vi "CLD 13 Flow Rates Solution.vi"() -> ()   [LabVIEW 2014]
doc: "CLD-Lösung 13. Ereignisgesteuerte Zustandsautomatenarchitektur. Die Reihenfolge der Schritte richtet sich nach den Benutzereingaben."
uses:
  CLD 13 State Machine Enum.ctl
  CLD 13 Data Cluster.ctl
  CLD 13 timer Enum.ctl
panel:
  out "Fehler (Ausgang)":errorcluster
  in  "Fehler (Eingang, kein Fehler)":errorcluster
  out "Durchflussmesser":i8(knob) scale=-20.0..20.0 scale format="%_2f"
  in  "Applikation stoppen":bool
  in  "Durchfluss stoppen":bool
  out "Verstrichene Zeit":dbl format="%#.1g"
  out "Flussrate":dbl
  in  "Flussratenänderung":i8(slide) min=-2 max=2 step=1 scale=-2.0..2.0
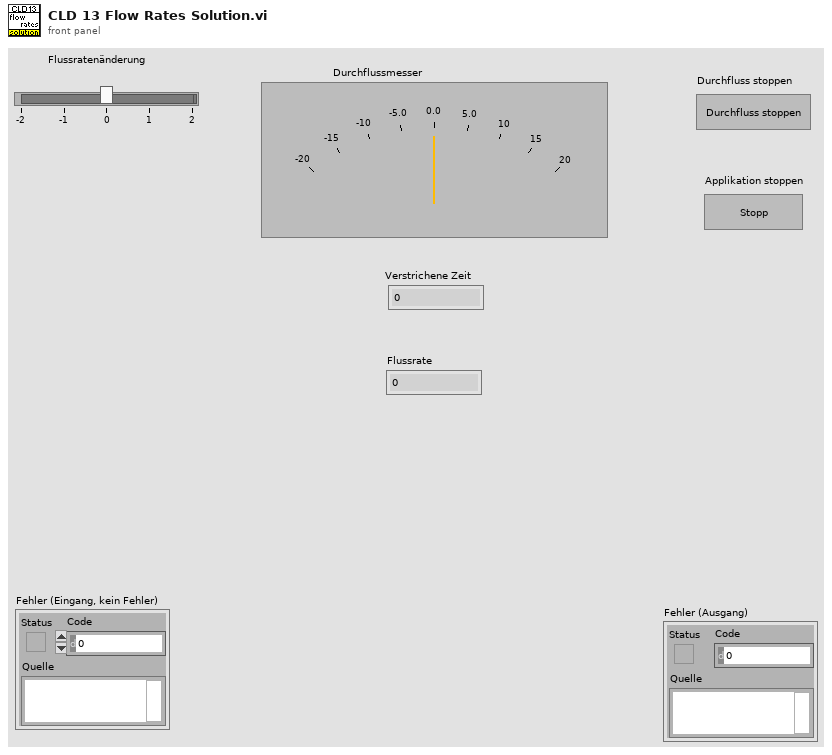
[diagram p1: front panel]
types:
  T1 = typedef "CLD 13 Data Cluster.ctl" = cluster{"Flussratenänderung":i8, "Flussrate":i8}
  T2 = typedef "CLD 13 State Machine Enum.ctl" = enum16{"Initialisieren", "Ruhezustand", "Durchfluss stoppen", "Prozess"}
  T3 = typedef "CLD 13 timer Enum.ctl" = enum16{"Starten", "Lesen"}
  T4 = cluster{"Status":bool, "Code":i32, "Quelle":string}
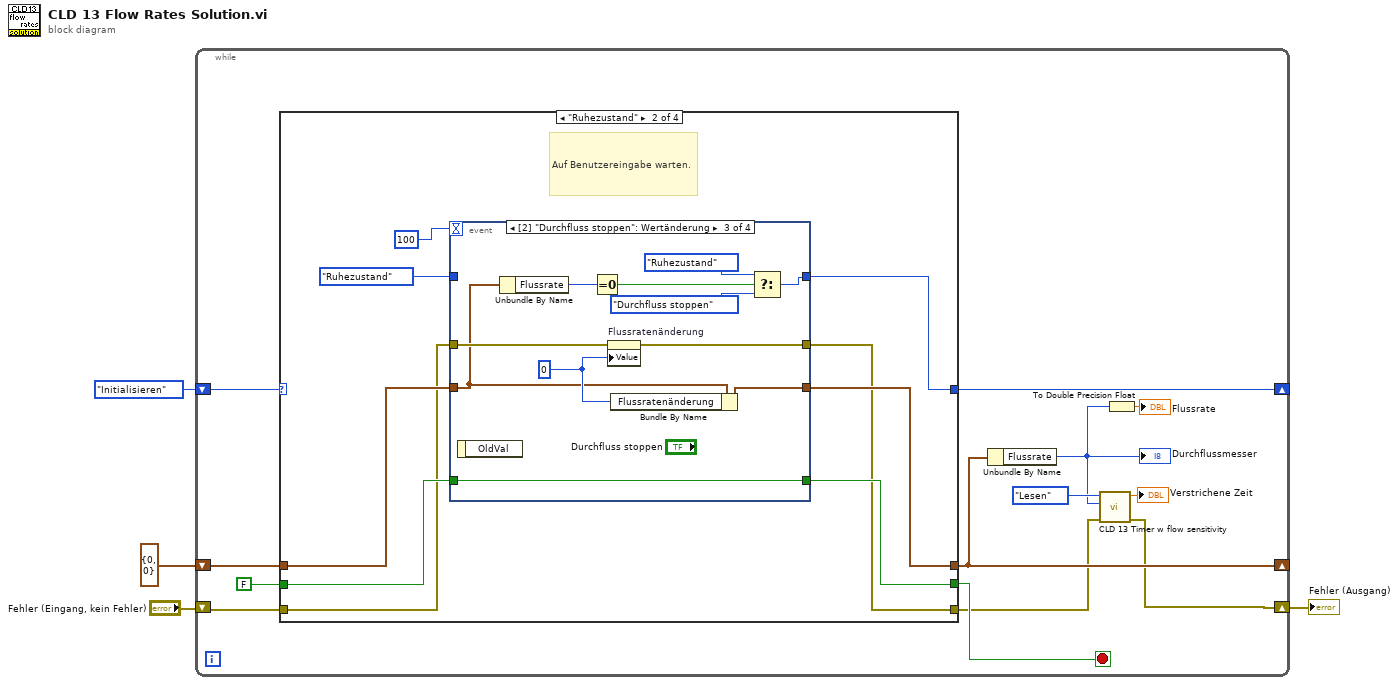
[diagram p0: block diagram]
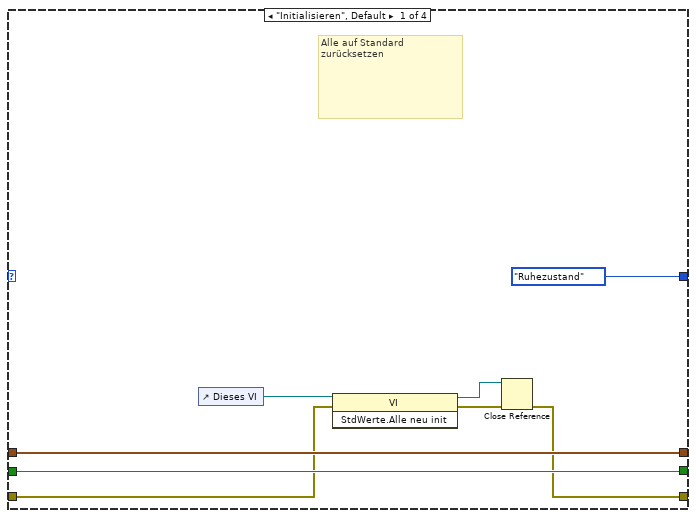
[diagram p2: hidden frame]
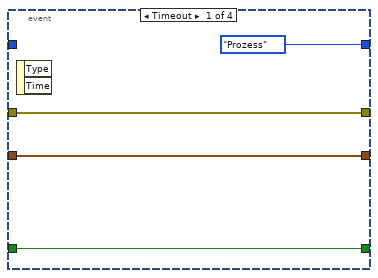
[diagram p3: hidden frame]
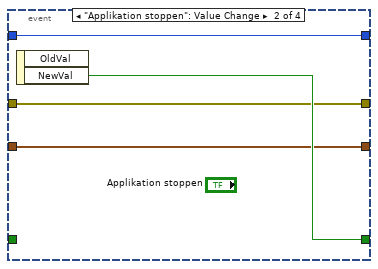
[diagram p4: hidden frame]
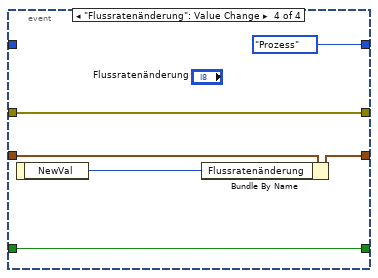
[diagram p5: hidden frame]
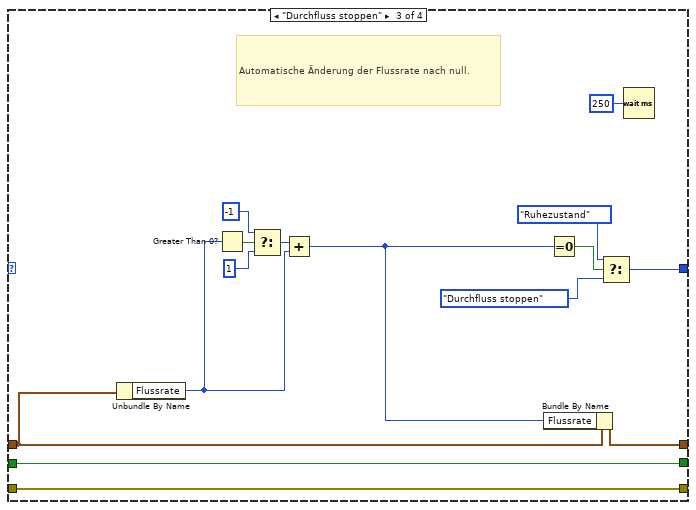
[diagram p6: hidden frame]
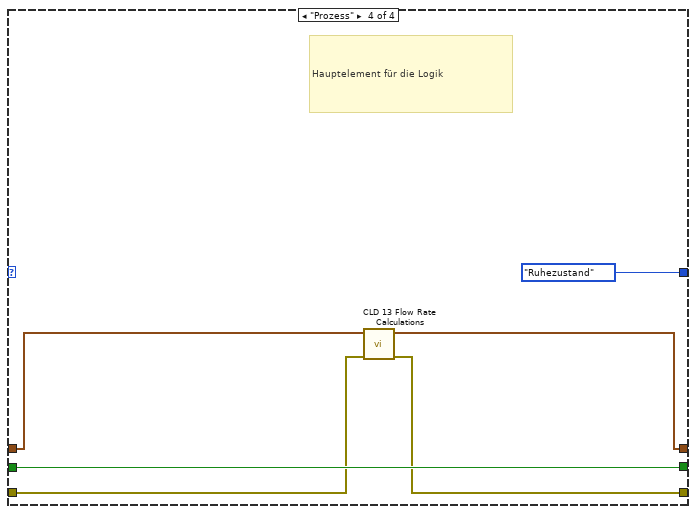
[diagram p7: hidden frame]
diagram:
  n1 = while {
    shift-right: [w14] -> _
    shift-left: CLD_13_State_Machine_Enum."Initialisieren" ("Enum") -> [w17]
    shift-right: [w12] -> _
    shift-left: T1 {"Flussratenänderung"=0, "Flussrate"=0} -> [w13]
    shift-right: [w7] -> w2
    shift-left: "Fehler (Eingang, kein Fehler)" -> [w10]
    stop <- w16 stop-if-true
    n2 = case shown="\"Ruhezustand\"" w17 {
      tunnel: [w25 w33 w74 w80] -> w16
      tunnel: FALSE -> [w25 w34 w74 w80]
      tunnel: [CLD_13_State_Machine_Enum."Ruhezustand" ("Enum") w30 w64 CLD_13_State_Machine_Enum."Ruhezustand" ("Enum")] -> w14
      tunnel: w13 -> [w23 w32 w73 w79]
      tunnel: [w23 w31 w72 w78] -> w12
      tunnel: [w18 w26 w62 w75] -> w8
      tunnel: w10 -> [w19 w27 w62 w76]
      frame "Initialisieren", Default {
        # "Alle auf Standard zurücksetzen"
        n3 = control-ref of="Dieses VI"() -> (w20:refnum<vi>)
        n4 = invoke on="Invoke Node" class="VI" method="StdWerte.Alle neu init"(reference=w20, error in=w19) -> (reference out=w21:refnum<vi>, error out=w22:errorcluster)  [unwired: 1 in, 1 out]
        n5 = Close Reference(reference=w21, error in (no error)=w22) -> (error out=w18:errorcluster)
      }
      frame "Ruhezustand" {
        # "Auf Benutzereingabe warten."
        n6 = event shown="[2] \"Durchfluss stoppen\": Wertänderung" {
          selector: _ -> [_ _ _ _]
          dyn-events: _ -> [_ _ _ _]
          timeout: 100 -> [_ _ _ _]
          tunnel: w34 -> [w38 _ w53 w58]
          tunnel: [w38 w42 w53 w58] -> w33
          tunnel: w32 -> [w37 w41 w48 w55]
          tunnel: [w37 w41 w50 w59] -> w31
          tunnel: [CLD_13_State_Machine_Enum."Prozess" ("Enum") w40 w43 CLD_13_State_Machine_Enum."Prozess" ("Enum")] -> w30
          tunnel: CLD_13_State_Machine_Enum."Ruhezustand" ("Enum") -> [_ w40 _ _]
          tunnel: w27 -> [w35 w39 w52 w54]
          tunnel: [w35 w39 w51 w54] -> w26
          event Timeout {
            n7 = event-data() -> ()  [unwired: 1 in, 2 out]
          }
          event "Applikation stoppen": Value Change {
            n8 = event-data() -> ("NewVal"=w42:bool)  [unwired: 1 in, 1 out]
          }
          event "Durchfluss stoppen": Value Change {
            w49 = i8 0 ("Flussrate")
            n9 = event-data() -> ()  [unwired: 1 in, 1 out]
            n10 = Unbundle By Name(w48) -> ("Flussrate"=w47:i8)
            n11 = Equal To 0?(x=w47) -> (x = 0?=w46:bool)
            n12 = property on="Flussratenänderung" class="Schieber (strikt)"(error in=w52, "Value"=w49) -> (error out=w51:errorcluster)  [unwired: 1 in, 1 out]
            n13 = Bundle By Name(cluster=w48, "Flussratenänderung"=w49) -> (w50:T1)
            n14 = Select(t=CLD_13_State_Machine_Enum."Ruhezustand" ("Enum"), s=w46, f=CLD_13_State_Machine_Enum."Durchfluss stoppen" ("Enum")) -> (s? t:f=w43:T2)
          }
          event "Flussratenänderung": Value Change {
            n15 = event-data() -> ("NewVal"=w56:i8)  [unwired: 1 in]
            n16 = Bundle By Name(cluster=w55, "Flussratenänderung"=w56) -> (w59:T1)
          }
        }
      }
      frame "Durchfluss stoppen" {
        # "Automatische Änderung der Flussrate nach null."
        n17 = Unbundle By Name(w73) -> ("Flussrate"=w61:i8)
        n18 = Greater Than 0?(x=w61) -> (x > 0?=w71:bool)
        n19 = Select(t=i8 -1 ("Flussrate"), s=w71, f=i8 1 ("Flussrate")) -> (s? t:f=w70:i8)
        n20 = Add(x=w70, y=w61) -> (x+y=w60:i8)
        n21 = Bundle By Name(cluster=w73, "Flussrate"=w60) -> (w72:T1)
        n22 = Equal To 0?(x=w60) -> (x = 0?=w65:bool)
        n23 = Select(t=CLD_13_State_Machine_Enum."Ruhezustand" ("Enum"), s=w65, f=CLD_13_State_Machine_Enum."Durchfluss stoppen" ("Enum")) -> (s? t:f=w64:T2)
        n24 = Wait (ms)(milliseconds to wait=u32 250 ("Zu wartende ms")) -> ()  [unwired: 1 out]
      }
      frame "Prozess" {
        # "Hauptelement für die Logik"
        n25 = call "CLD 13 Flow Rate Calculations.vi"("Fehler (Eingang)"=w76, "Cluster (Eingang)"=w79) -> ("Fehler (Ausgang)"=w75:T4, "Cluster (Ausgang)"=w78:T1)  [unwired: 8 in]
      }
    }
    n26 = Unbundle By Name(w12) -> ("Flussrate"=w5:i8)
    "Durchflussmesser" <- w5
    n27 = call "CLD 13 Timer w flow sensitivity.vi"("Fehler (Eingang)"=w8, "Flussrate"=w5, "Timer-Enum"=CLD_13_timer_Enum."Lesen") -> ("Fehler (Ausgang)"=w7:T4, "Verstrichene Zeit"=→"Verstrichene Zeit":dbl)  [unwired: 7 in]
    n28 = To Double Precision Float(number=w5) -> (double precision float=→"Flussrate":dbl)
  }
  "Fehler (Ausgang)" <- w2
